vi "Move Group Along Line.vi"(4 "error in (no error)":errorcluster, 5 "Position (0 units)":dbl[](array[numeric]), 6 "Group Number (1)":i32=1 min=1, 7 "VISA resource name":refnum<visa-resource-name>) -> (0 "error out":errorcluster, 3 "VISA resource name out":refnum<visa-resource-name>)   [LabVIEW 2014, in "Newport ESP301.lvlib"]
doc: "This command initiates motion of a group along a line. It causes all axes assigned to the group to move with predefined vectorial (tangential) velocity, acceleration and deceleration along a line. A trapezoid velocity profile is employed when vectorial jerk is set to zero. Otherwise, an S-curve velocity profile is employed.\nIf this command is received while a group move is in progress, the new command gets enqueued into a “via point” buffer. Please refer Advanced Capabilities section for a detailed description of via point buffer implementation. The enqueued commands get executed on a FIFO basis when the move already in progress has reached its destination. The group does not come to a stop at the end of last move. Instead, there will be a smooth transition to the new move command, just as if it were one compound move (combination of multiple moves).\n<B>Note:</B> The transition from last move to new move will be smooth if tangential velocity at the end of last move is the same as that at the beginning of new move."
uses:
  Newport ESP301.lvlib
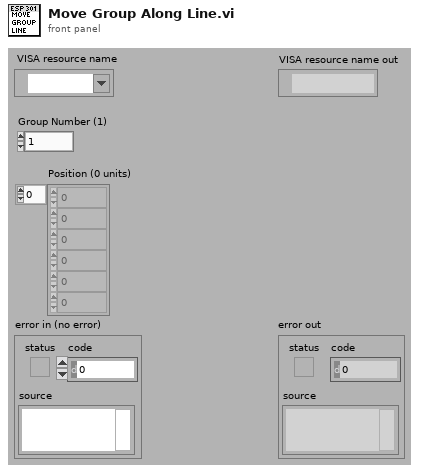
[diagram p1: front panel]
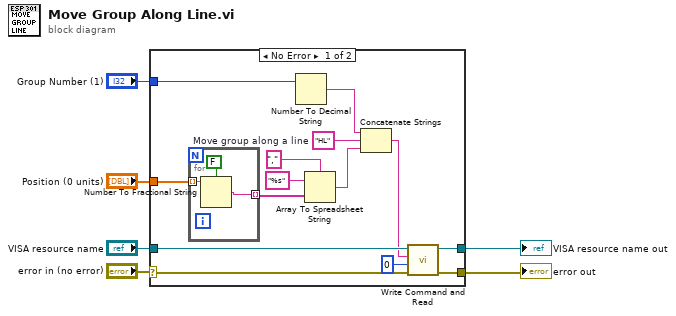
[diagram p0: block diagram]
diagram:
  n1 = case shown="No Error" "error in (no error)" {
    selector: "error in (no error)" -> [w17 w25]
    tunnel: [w19 w25] -> w6
    tunnel: "VISA resource name" -> [w20 w24]
    tunnel: [w18 w24] -> w5
    tunnel: "Group Number (1)" -> [w13 _]
    tunnel: "Position (0 units)" -> [w11 _]
    frame No Error {
      w16 = "HL"  # Move group along a line
      n2 = for {
        tunnel: w11 -> [w23] mode=indexing
        tunnel: [w21] -> w10 mode=indexing
        n3 = Number To Fractional String(use system decimal point (T)=FALSE ("utiliser le séparateur décimal du système (V)"), number=w23) -> (F-format string=w21:string)  [unwired: 2 in]
      }
      n4 = Number To Decimal String(number=w13) -> (decimal integer string=w15:string)  [unwired: 1 in]
      n5 = Array To Spreadsheet String(delimiter (Tab)="," ("chaîne"), array=w10, 3:"%s" ("format string")) -> (spreadsheet string=w7:string)
      n6 = Concatenate Strings(w15, w16, w7) -> (w14:string)
      n7 = call "Write Command and Read.vi"("error in (no error)"=w17, "Bytes to read (100)"=u32 0, "Command"=w14, "VISA resource name"=w20) -> ("error out"=w19:errorcluster, "VISA resource name out"=w18:refnum<visa-resource-name>)  [unwired: 3 in, 1 out]
    }
    frame Error {
    }
  }
  "error out" <- w6
  "VISA resource name out" <- w5
